vi "NMRFMTCP5.vi"() -> ()   [LabVIEW 2013]
uses:
  <vilib>/Analysis/2dsp.llb/Power Spectrum (DBL).vi
  kleinjan/MKS/Global - Pressure & Flow.vi
  <vilib>/Analysis/NI_AALBase.lvlib
  <vilib>/Analysis/NI_AALPro.lvlib
panel:
  out "initphase":dbl=2.08 format="%#_13g"
  out "inittune":dbl=1.244 format="%#_13g"
  in  "Save Tune":bool
  in  "Tune?":bool
  out "Date / Time":string="12/5/2017 4:21:17 PM"
  in  "Stop Run":bool=TRUE
  out "He readback":bool
  in  "Prompt?":bool
  out "He temp (K)":sgl=2.13326 format="%.3f"
  out "He press (torr)":sgl=33.89 format="%.3f"
  in  "NMR Channel Select":string(combo)="Tune2.csv"
  out "Color Box":u32(colorbox)=16775210
  out "Measurement":enum16{"TEQ", "POL", "QCV"}(ring)
  in  "VME IP Address":string="192.168.0.4"
  out "FFT Vrms":dbl[](graph)=[0.00665461346633416, 0.0013184205958180774, 0.00032493347048972255, 0.00014777056763622272, 9.381274661705268e-05, 5.694492256043897e-05, 2.4602515151070093e-05, 2.4735928736174615e-05, 1.7238804666774456e-05, 1.8474256556130103e-05, 3.88140821584203e-06, 1.2602440301653875e-05, 8.328027067854474e-06, 9.714098656211597e-06, 9.591073826282002e-06, 1.8400610475153133e-06, 3.891822160858666e-06, 7.42860213832651e-07, 4.960531568911141e-06, 1.0357752920077204e-05, 8.821106198975682e-06, 4.297248862721329e-06, 6.756736241898357e-06, 1.1507829286001889e-05, 6.285430593231241e-06, 5.699497906089993e-06, 4.826883317592869e-06, 1.0954894980259898e-05, 8.548451061857287e-06, 8.288312118460071e-07, 3.496252158688967e-06, 4.446519758691104e-06, 1.1272471497109705e-06, 2.984287855648866e-06, 4.4013212799680506e-06, 2.7233378655836314e-06, 8.028051828202549e-06, 2.7179961404271994e-06, 2.741222097162825e-06, 8.272000128623847e-06, 5.062564520990176e-06, 5.342721918389221e-06, 4.655150514690805e-06, 3.7370639785257395e-06, 2.136800574890996e-06, 1.8266511330512507e-06, 1.284347857617383e-06, 2.0013558699868966e-06, 1.2042755969189114e-06, 6.058284222290214e-06, 7.389298504405541e-06, 2.77971188428063e-06, 7.697014337872333e-06, 4.09073583086401e-06, 3.1016991758581816e-06, 5.282645474294868e-07, 3.246106814596551e-06, 1.5964327844448069e-06, 3.2408118302431348e-06, 1.9033736338368444e-06, 6.683740481872343e-06, 2.6688168177704896e-06, 1.8040110478604363e-06, 5.689652571752047e-07, 4.566365523818322e-06, 7.67651980126649e-06, 3.6261391438622403e-06, 1.962113938019778e-06, 1.9575774542411484e-06, 6.113330203835039e-06, 4.837593307405045e-06, 1.5646329065944149e-06, 1.9642799364610824e-06, 5.344757267984994e-06, 1.4903732944971783e-06, 2.3253986011212398e-06, 3.505294515533926e-06, 1.2861248933475453e-06, 3.1756847203363983e-06, 5.210539488954998e-06, 5.873764257939144e-06, 1.488838318327932e-06, 3.4258096560470588e-06, 4.6561579367461355e-06, 3.3604761794694807e-06, 5.166120910958792e-06, 4.852422673140418e-06, 6.413144484541961e-06, 2.3873635432332113e-06, 4.815191295361827e-06, 4.599370623864332e-06, 4.533502118577405e-06, 4.251902968067585e-06, 1.1589988767519234e-06, 2.3203344894473095e-07, 4.066434795829476e-06, 3.46145032312765e-06, 3.2547198313791895e-06, 2.1219983709150387e-06, 4.495545878631818e-06, 3.110572503955211e-07, 1.589264311064526e-06, 3.3006546489564546e-06, 3.239107109046435e-06, 1.956587615390749e-06, 1.0821609125242872e-06, 4.18172944578455e-06, 3.4672825501217612e-06, 3.0604596728264873e-06, 2.249802101656082e-06, 3.6396234355254457e-06, 1.9148250175480704e-06, 6.100574262898342e-06, 2.040562898958206e-06, 3.681543145664905e-06, 6.36570977326168e-06, 3.978270510621126e-06, 2.9167261060330305e-06, 4.596371371759104e-06, 1.7082086474587407e-06, 1.0983887595677434e-06, 1.6801012803857932e-06, 1.8127834158020698e-06, 4.439505513519553e-06, 1.6592215036724682e-06, 2.5343701898196556e-06, 6.407230283423339e-06, 2.878137385486302e-06, 1.0359403307825742e-06, 3.401981562355416e-06, 4.492298826850195e-06, 4.244045593799213e-06, 2.4547652511595895e-06, 2.287980497906362e-06, 4.064951112754048e-06, 1.0150896867566275e-05, 5.111642196581524e-06, 2.7553627360277643e-06, 5.09313899121079e-07, 5.768699698084646e-06, 3.2661863048088682e-06, 5.576911536051898e-06, 1.3992030895115723e-06, 5.793480137064482e-07, 4.167273754327372e-06, 2.803767211933649e-06, 1.290492108720642e-06, 1.4073374274672208e-06, 2.2326186185191207e-06, 2.361435359052297e-06, 1.1075042044185725e-06, 9.822428126647478e-07, 1.4402015890510517e-06, 3.4799861239118846e-06, 6.876662204989774e-07, 2.9528766955207207e-06, 3.987038034312176e-06, 2.4223930611358374e-06, 2.4859113073777655e-06, 2.676948548044152e-06, 3.001197081641741e-06, 1.3437660563498952e-06, 4.530463234261475e-06, 3.5418577344012663e-06, 9.285218882268811e-07, 2.448991731608343e-06, 4.237615365541793e-06, 9.437753499711396e-06, 4.733601144522179e-06, 1.1993912833596027e-06, 4.592206510692074e-06, 1.6445086805399158e-06, 2.28625361595349e-06, 2.7657675123967644e-06, 4.727937271980666e-06, 1.1243035877642484e-06, 2.963405459320666e-06, 2.4221501912349967e-06, 4.3573020759701795e-06, 6.067249298625184e-06, 4.689337884831793e-06, 1.5356012824001038e-06, 4.493628958545829e-06, 2.750405264990747e-06, 1.803652857072422e-06, 5.477945487956627e-06, 4.241114523214695e-06, 3.110895691004747e-06, 4.4944025519747775e-06, 1.9660519605861145e-06, 3.642406557905753e-06, 3.6774228456584596e-06, 1.6639882217832455e-06, 6.260045262480856e-07, 4.334327770598918e-06, 5.214873834167074e-06, 1.730017114321754e-06, 1.93737641122103e-06, 3.517495286731861e-06, 1.7057836116701932e-06, 3.185318567505982e-06, 3.185318567505982e-06, 1.7057836116701932e-06, 3.517495286731861e-06, 1.93737641122103e-06, 1.730017114321754e-06, 5.214873834167074e-06, 4.334327770598918e-06, 6.260045262480856e-07, 1.6639882217832455e-06, 3.6774228456584596e-06, 3.642406557905753e-06, 1.9660519605861145e-06, 4.4944025519747775e-06, 3.110895691004747e-06, 4.241114523214695e-06, 5.477945487956627e-06, 1.803652857072422e-06, 2.750405264990747e-06, 4.493628958545829e-06, 1.5356012824001038e-06, 4.689337884831793e-06, 6.067249298625184e-06, 4.3573020759701795e-06, 2.4221501912349967e-06, 2.963405459320666e-06, 1.1243035877642484e-06, 4.727937271980666e-06, 2.7657675123967644e-06, 2.28625361595349e-06, 1.6445086805399158e-06, 4.592206510692074e-06, 1.1993912833596027e-06, 4.733601144522179e-06, 9.437753499711396e-06, 4.237615365541793e-06, 2.448991731608343e-06, 9.285218882268811e-07, 3.5418577344012663e-06, 4.530463234261475e-06, 1.3437660563498952e-06, 3.001197081641741e-06, 2.676948548044152e-06, 2.4859113073777655e-06, 2.4223930611358374e-06, 3.987038034312176e-06, 2.9528766955207207e-06, 6.876662204989774e-07, 3.4799861239118846e-06, 1.4402015890510517e-06, 9.822428126647478e-07, 1.1075042044185725e-06, 2.361435359052297e-06, 2.2326186185191207e-06, 1.4073374274672208e-06, 1.290492108720642e-06, 2.803767211933649e-06, 4.167273754327372e-06, 5.793480137064482e-07, 1.3992030895115723e-06, 5.576911536051898e-06, 3.2661863048088682e-06, 5.768699698084646e-06, 5.09313899121079e-07, 2.7553627360277643e-06, 5.111642196581524e-06, 1.0150896867566275e-05, 4.064951112754048e-06, 2.287980497906362e-06, 2.4547652511595895e-06, 4.244045593799213e-06, 4.492298826850195e-06, 3.401981562355416e-06, 1.0359403307825742e-06, 2.878137385486302e-06, 6.407230283423339e-06, 2.5343701898196556e-06, 1.6592215036724682e-06, 4.439505513519553e-06, 1.8127834158020698e-06, 1.6801012803857932e-06, 1.0983887595677434e-06, 1.7082086474587407e-06, 4.596371371759104e-06, 2.9167261060330305e-06, 3.978270510621126e-06, 6.36570977326168e-06, 3.681543145664905e-06, 2.040562898958206e-06, 6.100574262898342e-06, 1.9148250175480704e-06, 3.6396234355254457e-06, 2.249802101656082e-06, 3.0604596728264873e-06, 3.4672825501217612e-06, 4.18172944578455e-06, 1.0821609125242872e-06, 1.956587615390749e-06, 3.239107109046435e-06, 3.3006546489564546e-06, 1.589264311064526e-06, 3.110572503955211e-07, 4.495545878631818e-06, 2.1219983709150387e-06, 3.2547198313791895e-06, 3.46145032312765e-06, 4.066434795829476e-06, 2.3203344894473095e-07, 1.1589988767519234e-06, 4.251902968067585e-06, 4.533502118577405e-06, 4.599370623864332e-06, 4.815191295361827e-06, 2.3873635432332113e-06, 6.413144484541961e-06, 4.852422673140418e-06, 5.166120910958792e-06, 3.3604761794694807e-06, 4.6561579367461355e-06, 3.4258096560470588e-06, 1.488838318327932e-06, 5.873764257939144e-06, 5.210539488954998e-06, 3.1756847203363983e-06, 1.2861248933475453e-06, 3.505294515533926e-06, 2.3253986011212398e-06, 1.4903732944971783e-06, 5.344757267984994e-06, 1.9642799364610824e-06, 1.5646329065944149e-06, 4.837593307405045e-06, 6.113330203835039e-06, 1.9575774542411484e-06, 1.962113938019778e-06, 3.6261391438622403e-06, 7.67651980126649e-06, 4.566365523818322e-06, 5.689652571752047e-07, 1.8040110478604363e-06, 2.6688168177704896e-06, 6.683740481872343e-06, 1.9033736338368444e-06, 3.2408118302431348e-06, 1.5964327844448069e-06, 3.246106814596551e-06, 5.282645474294868e-07, 3.1016991758581816e-06, 4.09073583086401e-06, 7.697014337872333e-06, 2.77971188428063e-06, 7.389298504405541e-06, 6.058284222290214e-06, 1.2042755969189114e-06, 2.0013558699868966e-06, 1.284347857617383e-06, 1.8266511330512507e-06, 2.136800574890996e-06, 3.7370639785257395e-06, 4.655150514690805e-06, 5.342721918389221e-06, 5.062564520990176e-06, 8.272000128623847e-06, 2.741222097162825e-06, 2.7179961404271994e-06, 8.028051828202549e-06, 2.7233378655836314e-06, 4.4013212799680506e-06, 2.984287855648866e-06, 1.1272471497109705e-06, 4.446519758691104e-06, 3.496252158688967e-06, 8.288312118460071e-07, 8.548451061857287e-06, 1.0954894980259898e-05, 4.826883317592869e-06, 5.699497906089993e-06, 6.285430593231241e-06, 1.1507829286001889e-05, 6.756736241898357e-06, 4.297248862721329e-06, 8.821106198975682e-06, 1.0357752920077204e-05, 4.960531568911141e-06, 7.42860213832651e-07, 3.891822160858666e-06, 1.8400610475153133e-06, 9.591073826282002e-06, 9.714098656211597e-06, 8.328027067854474e-06, 1.2602440301653875e-05, 3.88140821584203e-06, 1.8474256556130103e-05, 1.7238804666774456e-05, 2.4735928736174615e-05, 2.4602515151070093e-05, 5.694492256043897e-05, 9.381274661705268e-05, 0.00014777056763622272, 0.00032493347048972255, 0.0013184205958180774]
  out "Raw NMR Graph / Ave":cluster{dbl, "Step Width (MHz)":dbl, dbl[][]}(graph)={212.6, "Step Width (MHz)"=0.002, []}
  in  "R&S GPIB Addr (28)":refnum<visa-resource-name>="GPIB1::28::INSTR"
  out "Pedestal (V)":dbl=0.007879166666666666 format="%_2g"
  in  "Open Global Panel":bool
  out "Peak center (MHz)":sgl=212.61032 format="%.3f"
  out "Telnet error out":errorcluster
  out "+3.3V supply":dbl=3.294 format="%_4g"
  out "Temp (C)":dbl=25.0 format="%_4g"
  out "RF level OK":bool=TRUE
  out "Peak area (V-MHz)":sgl=-0.97693336 format="%.5f"
  out "# Good Spectra":i32=1000
  out "Pedestal volts OK":bool=TRUE
  out "Sweep #":i32=88
  out "1st Sweep":bool
  out "ADC volts OK":bool=TRUE
  out "Peak Height Distribution":cluster{"Y":dbl[], "Y":dbl[]}[](graph)=[{"Y"=[0.003985987500000001, 0.0039929625000000015, 0.003999937500000002, 0.004006912500000002, 0.004013887500000001, 0.0040208625000000015, 0.004027837500000002, 0.004034812500000002, 0.004041787500000001, 0.0040487625000000015, 0.004055737500000002, 0.004062712500000002, 0.004069687500000001, 0.0040766625000000015, 0.004083637500000002, 0.004090612500000001, 0.004097587500000001, 0.0041045625000000014, 0.004111537500000002, 0.004118512500000001, 0.004125487500000001, 0.004132462500000001, 0.004139437500000002, 0.004146412500000001, 0.004153387500000001, 0.004160362500000001, 0.004167337500000002, 0.004174312500000001, 0.004181287500000001, 0.004188262500000001, 0.004195237500000002, 0.004202212500000001, 0.004209187500000001, 0.004216162500000001, 0.0042231375000000015, 0.004230112500000001, 0.004237087500000001, 0.004244062500000001, 0.004251037500000001, 0.004258012500000001, 0.004264987500000001, 0.004271962500000001, 0.004278937500000001, 0.004285912500000001, 0.004292887500000001, 0.004299862500000001, 0.004306837500000001, 0.004313812500000001, 0.004320787500000001, 0.004327762500000001, 0.004334737500000001, 0.004341712500000001, 0.004348687500000001, 0.004355662500000001, 0.0043626375000000005, 0.004369612500000001, 0.004376587500000001, 0.004383562500000001, 0.0043905375000000005, 0.004397512500000001, 0.004404487500000001, 0.004411462500000001, 0.0044184375000000005, 0.004425412500000001, 0.004432387500000001, 0.0044393625, 0.0044463375000000005, 0.004453312500000001, 0.004460287500000001, 0.0044672625, 0.0044742375000000004, 0.004481212500000001, 0.004488187500000001, 0.0044951625, 0.0045021375, 0.004509112500000001, 0.004516087500000001, 0.0045230625, 0.0045300375, 0.004537012500000001, 0.004543987500000001, 0.0045509625, 0.0045579375, 0.004564912500000001, 0.004571887500000001, 0.0045788625, 0.0045858375, 0.0045928125000000005, 0.004599787500000001, 0.0046067625, 0.0046137375, 0.0046207125000000005, 0.0046276875, 0.0046346625, 0.0046416375, 0.0046486125000000005, 0.0046555875, 0.0046625625, 0.0046695375, 0.0046765125000000005], "Y"=[1.0, 0.0, 0.0, 0.0, 0.0, 0.0, 0.0, 0.0, 2.0, 1.0, 0.0, 0.0, 0.0, 1.0, 4.0, 3.0, 3.0, 1.0, 0.0, 8.0, 2.0, 8.0, 8.0, 3.0, 2.0, 12.0, 12.0, 12.0, 2.0, 17.0, 13.0, 11.0, 11.0, 17.0, 19.0, 14.0, 17.0, 24.0, 13.0, 17.0, 14.0, 22.0, 21.0, 25.0, 26.0, 26.0, 23.0, 21.0, 29.0, 18.0, 25.0, 31.0, 24.0, 45.0, 24.0, 20.0, 29.0, 22.0, 19.0, 23.0, 17.0, 8.0, 13.0, 18.0, 24.0, 12.0, 22.0, 18.0, 8.0, 8.0, 10.0, 9.0, 13.0, 8.0, 8.0, 6.0, 5.0, 5.0, 4.0, 4.0, 4.0, 8.0, 3.0, 5.0, 3.0, 1.0, 1.0, 1.0, 3.0, 1.0, 1.0, 0.0, 1.0, 0.0, 0.0, 1.0, 0.0, 1.0, 0.0, 1.0]}]
  out "S/N":dbl=39.7281597738682 format="%_3g"
  out "Peak mean (V)":dbl=0.004333396666666667 format="%_3g"
  out "Pedestal Diff (V)":sgl=-0.00025166667 format="%.4f"
  out "Peak amp (V)":sgl=0.0031208333 format="%.4f"
  out "SMT error out":errorcluster
  out "Peak RMS (mV)":dbl=0.10907619913261185 format="%.3f"
  # "E1039 NMR Panel"
  # "Results"
  # "A\nv\ne\nr\na\ng\ne\ns"
  # "S\nw\ne\ne\np"
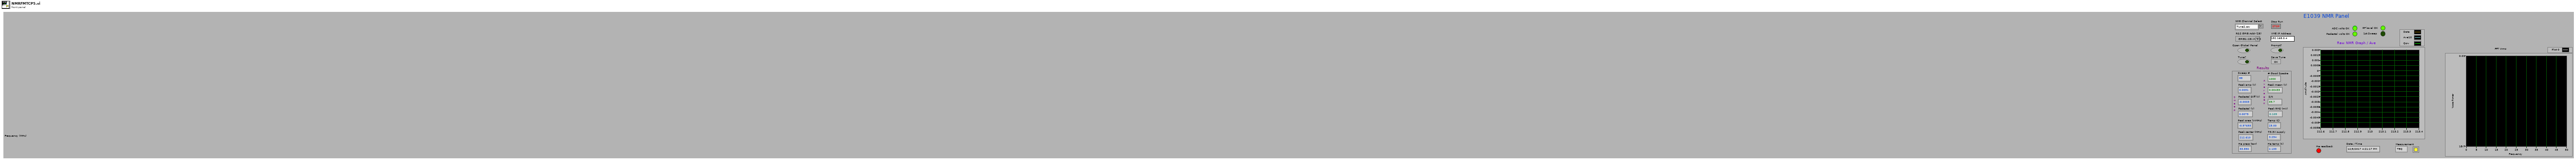
[diagram p1: front panel]
types:
  T1 = enum32{"Invalid", "Standard", "Closed", "Hidden", "Minimized", "Maximized"}
  T2 = enum32{"Bad", "Idle", "Run top level", "Running"}
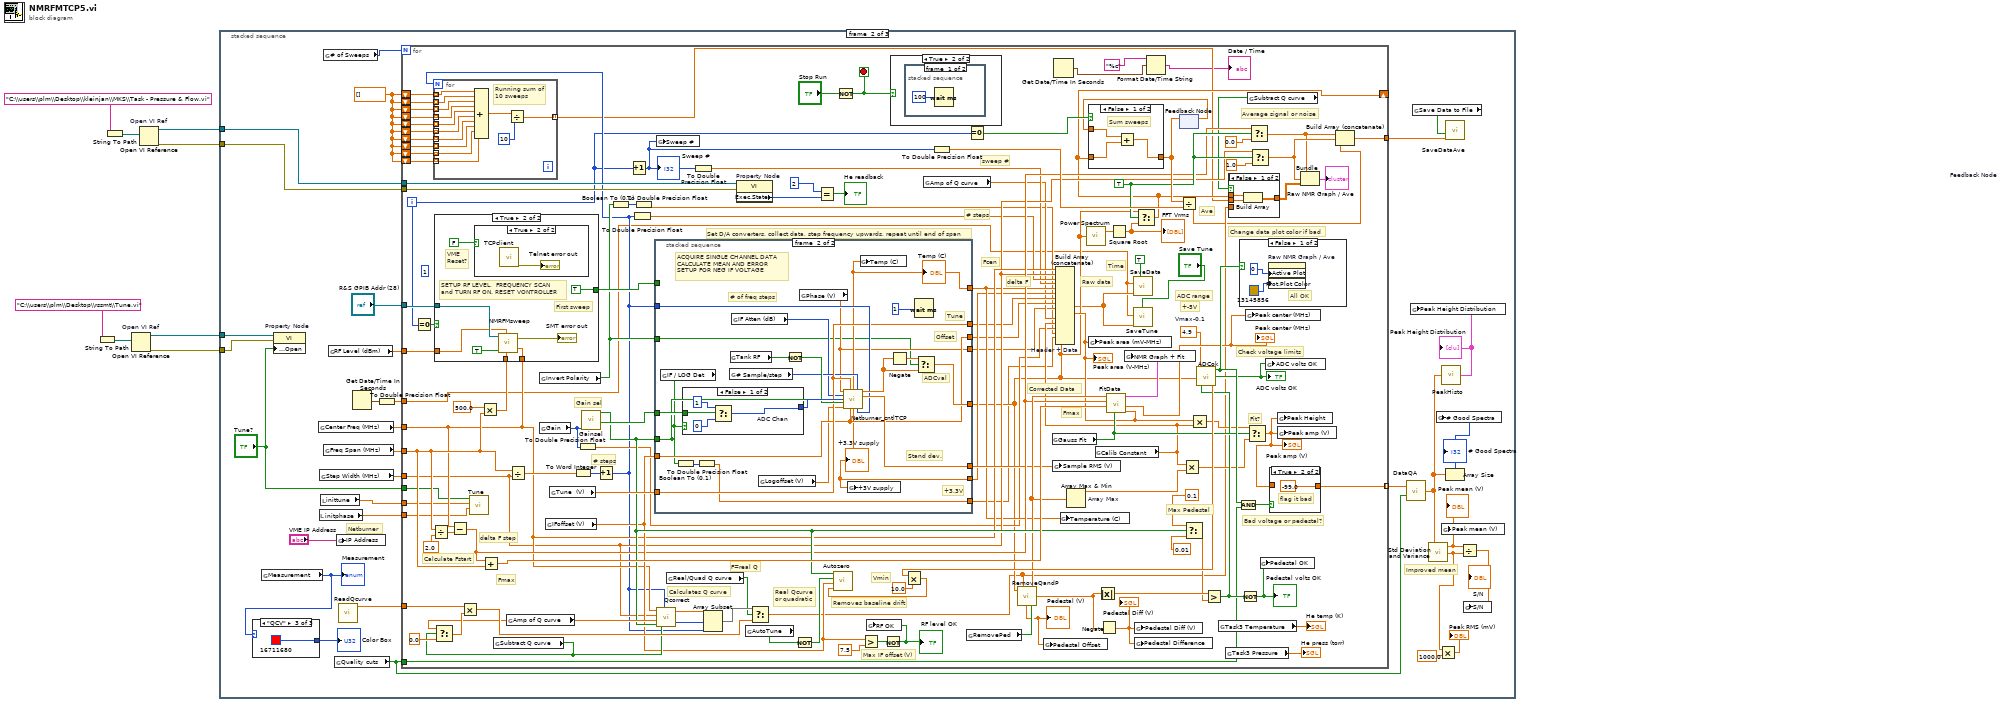
[diagram p0: block diagram]
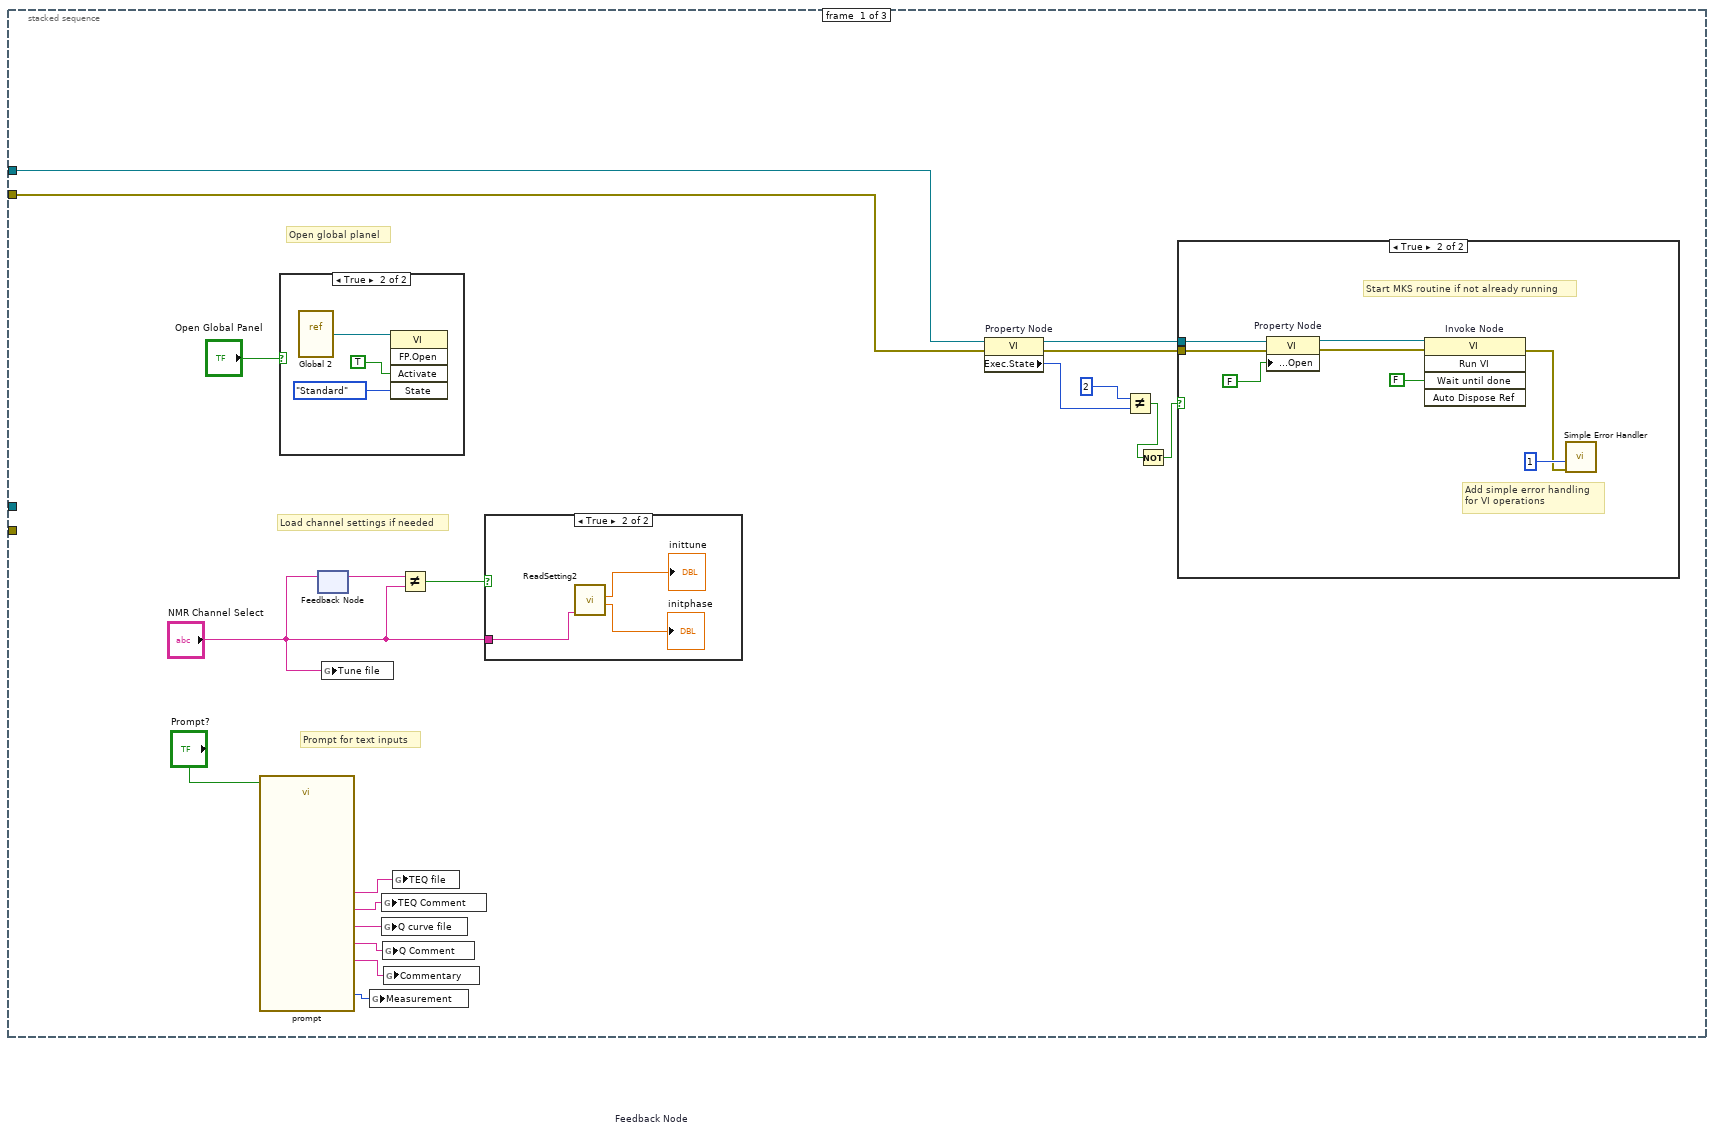
[diagram p2: hidden frame]
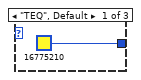
[diagram p6: hidden frame]
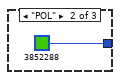
[diagram p7: hidden frame]
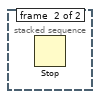
[diagram p9: hidden frame]
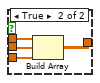
[diagram p10: hidden frame]
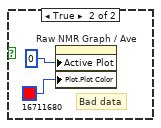
[diagram p12: hidden frame]
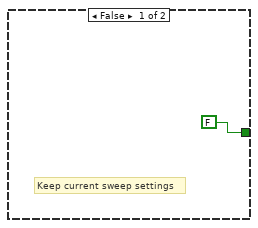
[diagram p14: hidden frame]
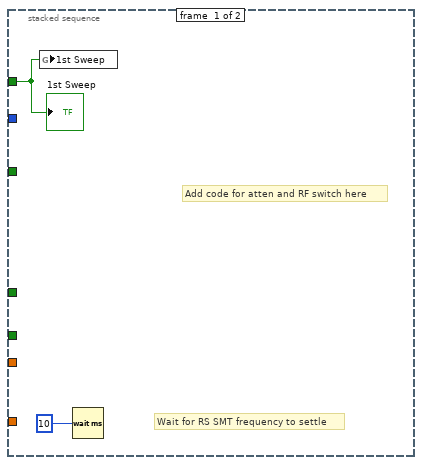
[diagram p16: hidden frame]
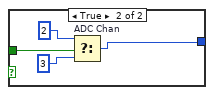
[diagram p17: hidden frame]
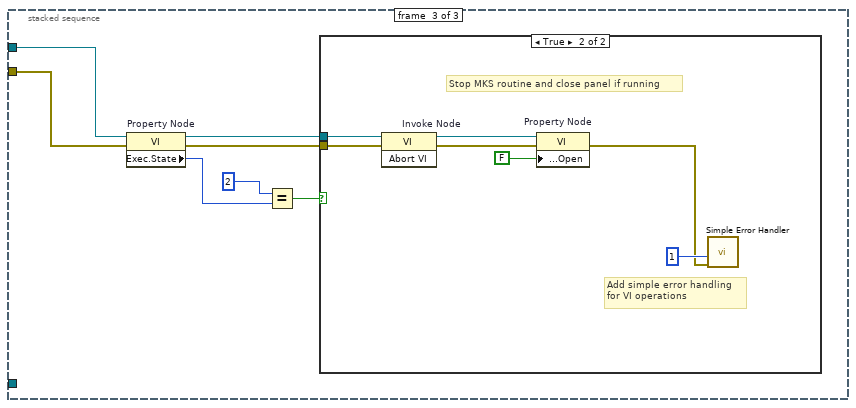
[diagram p18: hidden frame]
diagram:
  n1 = String To Path(string="C:\\users\\plm\\Desktop\\rssmt\\Tune.vi") -> (path=w4:path)
  n2 = String To Path(string="C:\\users\\plm\\Desktop\\kleinjan\\MKS\\Task - Pressure & Flow.vi") -> (path=w8:path)
  n3 = Open VI Reference "Open VI Ref"(vi path=w4) -> (vi reference=w2:refnum<vi>, error out=w1:errorcluster)  [unwired: 5 in]
  n4 = Open VI Reference "Open VI Ref"(vi path=w8) -> (vi reference=w5:refnum<vi>, error out=w6:errorcluster)  [unwired: 5 in]
  n5 = stacked-sequence {
    tunnel: w5 -> [w12 w49 w282]
    tunnel: w6 -> [w11 w48 w281]
    tunnel: w2 -> [_ w42 _]
    tunnel: w1 -> [_ w46 _]
    frame #0 {
      # "Prompt for text inputs"
      # "Load channel settings if needed"
      # "Open global planel"
      n6 = call "prompt.vi"("Enable"="Prompt?") -> ("Measurement"=w25:enum16{"TEQ", "POL", "QCV"}, "Run comment"=w24:string, "Q curve comment"=w23:string, "Q curve file"=w22:string, "TE Comment"=w21:string, "TE peak file"=w20:string)  [unwired: 11 in, 2 out]
      n7 = case shown="True" "Open Global Panel" {
        frame False {
        }
        frame True {
          n8 = vi-ref "Global 2.vi"() -> (w41:refnum<vi>)
          n9 = invoke class="VI" method="FP.Open"(reference=w41, "Activate"=TRUE, "State"=T1."Standard") -> ()  [unwired: 2 in, 5 out]
        }
      }
      n10 = feedback #1 "Feedback Node"() -> (w19:string)  [unwired: 1 in]
      n11 = feedback-in #1("NMR Channel Select") -> ()
      n12 = global write "Global 2.vi" "Tune file"("NMR Channel Select") -> ()
      n13 = global write "Global 2.vi" "Measurement"(w25) -> ()
      n14 = global write "Global 2.vi" "TEQ Comment"(w21) -> ()
      n15 = global write "Global 2.vi" "Q curve file"(w22) -> ()
      n16 = global write "Global 2.vi" "Q Comment"(w23) -> ()
      n17 = global write "Global 2.vi" "Commentary"(w24) -> ()
      n18 = global write "Global 2.vi" "TEQ file"(w20) -> ()
      n19 = Not Equal?(x=w19, y="NMR Channel Select") -> (x != y?=w18:bool)
      n20 = case shown="True" w18 {
        tunnel: "NMR Channel Select" -> [_ w38]
        frame False {
        }
        frame True {
          n21 = call "ReadSetting2.vi"("Data Filename"=w38) -> ("Phase"=→"initphase":dbl, "Tune"=→"inittune":dbl)  [unwired: 1 out]
        }
      }
      n22 = property on="Property Node" class="VI"(reference=w12, error in=w11) -> (reference out=w14:refnum<vi>, error out=w13:errorcluster, "Exec.State"=w15:T2)
      n23 = Not Equal?(x=2, y=w15) -> (x != y?=w10:bool)
      n24 = Not(x=w10) -> (.not. x?=w9:bool)
      n25 = case shown="True" w9 {
        tunnel: w14 -> [_ w32]
        tunnel: w13 -> [_ w31]
        frame False {
        }
        frame True {
          # "Start MKS routine if not already running"
          # "Add simple error handling\nfor VI operations"
          n26 = property on="Property Node" class="VI"(reference=w32, error in=w31, "Front Panel Window:Open"=FALSE ("Front Panel.Open")) -> (reference out=w30:refnum<vi>, error out=w29:errorcluster)
          n27 = invoke on="Invoke Node" class="VI" method="Run VI"(reference=w30, error in=w29, "Wait until done"=FALSE) -> (error out=w33:errorcluster)  [unwired: 2 in, 4 out]
          n28 = call <vilib>:"Simple Error Handler.vi"("type of dialog (OK msg:1)"=1, "error in (no error)"=w33) -> ()  [unwired: 3 in, 5 out]
        }
      }
    }
    frame #1 {
      w47 = dbl[] []
      # "Netburner"
      # "Improved mean"
      n29 = global read "Global 2.vi" "Measurement"() -> (w51:enum16{"TEQ", "POL", "QCV"})
      "Measurement" <- w51
      n30 = case shown="\"QCV\"" w51 {
        tunnel: [u32 16775210 ("Color Box 2") u32 3852288 ("Color Box 2") u32 16711680 ("Color Box 2")] -> w50
        frame "TEQ", Default {
        }
        frame "POL" {
        }
        frame "QCV" {
        }
      }
      "Color Box" <- w50
      n31 = property on="Property Node" class="VI"(reference=w42, error in=w46, "Front Panel Window:Open"="Tune?") -> ()  [unwired: 2 out]
      n32 = global read "Global 2.vi" "Center Freq (MHz)"() -> (w68:dbl)
      n33 = local read "initphase"() -> (w43:dbl)
      n34 = global read "Global 2.vi" "Step Width (MHz)"() -> (w66:dbl)
      n35 = local read "inittune"() -> (w44:dbl)
      n36 = global read "Global 2.vi" "# of Sweeps"() -> (w70:i32)
      n37 = global read "Global 2.vi" "Freq Span (MHz)"() -> (w67:dbl)
      n38 = global read "Global 2.vi" "RF Level (dBm)"() -> (w69:dbl)
      n39 = global read "Global 2.vi" "Quality cuts"() -> (w65:bool)
      n40 = global write "Global 2.vi" "IP Address"("VME IP Address") -> ()
      n41 = call "ReadQcurve.vi"() -> ("Array"=w56:dbl[])  [unwired: 2 in]
      n42 = Get Date/Time In Seconds() -> (seconds since 1Jan1904=w71:timestamp)
      n43 = To Double Precision Float(number=w71) -> (double precision float=w57:dbl)
      n44 = for {
        N: w70 -> [_]
        tunnel: [w198] -> w73 mode=indexing
        tunnel: w65 -> [w161]
        tunnel: w68 -> [w135]
        tunnel: w67 -> [w147]
        tunnel: w66 -> [w134]
        tunnel: "R&S GPIB Addr (28)" -> [w194]
        tunnel: w69 -> [w193]
        tunnel: w57 -> [w81]
        tunnel: w56 -> [w186]
        tunnel: [w151] -> w59
        tunnel: w49 -> [w108]
        tunnel: w48 -> [w107]
        shift-right: [w100] -> _
        shift-left: w47 -> [w99]
        shift-left: w47 -> [w90]
        shift-left: w47 -> [w98]
        shift-left: w47 -> [w97]
        shift-left: w47 -> [w96]
        shift-left: w47 -> [w95]
        shift-left: w47 -> [w94]
        shift-left: w47 -> [w93]
        shift-left: w47 -> [w92]
        shift-left: w47 -> [w91]
        tunnel: "Tune?" -> [w83]
        tunnel: w44 -> [w79]
        tunnel: w43 -> [w78]
        i -> [w88]
        stop <- w77 stop-if-true
        (unwired) 1
        w140 = TRUE
        w156 = 4.9  # Vmax-0.1
        # "Average signal or noise"
        # "Check voltage limits"
        # "Ave"
        # "Max Pedestal"
        # "Gain sel"
        # "F=real Q"
        # "Real Qcurve\nor quadratic"
        # "+-5V"
        # "Change data plot color if bad"
        # "Max IF offset (V)"
        # "Fmax"
        # "Fit?"
        # "Fmax"
        # "Time"
        # "Vmin"
        # "Raw data"
        # "Corrected Data"
        # "Fcen"
        # "delta F"
        # "# steps"
        # "ADC range"
        # "sweep #"
        # "Set D/A converters, collect data, step frequency upwards, repeat until end of span"
        # "Calculates Q curve"
        # "Removes baseline drift"
        # "Bad voltage or pedestal?"
        # "# steps"
        # "Calculate Fstart"
        # "delta F step"
        n45 = Equal To 0?(x=w88) -> (x = 0?=w200:bool)
        n46 = Divide(x=w147, y=sgl 2.0) -> (x/y=w204:dbl)
        n47 = Subtract(x=w135, y=w204) -> (x-y=w138:dbl)
        n48 = call "Tune.vi"("Init Phase V"=w78, "Init Tune V"=w79, "Tune"=w83) -> ()  [unwired: 9 in]
        n49 = Multiply(x=500.0, y=w147) -> (x*y=w146:dbl)
        n50 = case shown="True" w200 {
          tunnel: w135 -> [_ w245]
          tunnel: w146 -> [_ w246]
          tunnel: [FALSE TRUE] -> w199
          tunnel: w194 -> [_ w242]
          tunnel: w193 -> [_ w241]
          frame False {
            # "Keep current sweep settings"
          }
          frame True {
            # "VME\nReset?"
            # "First sweep"
            # "SETUP RF LEVEL,  FREQUENCY SCAN\nand TURN RF ON. RESET VONTROLLER"
            n51 = case shown="True" FALSE {
              frame False {
              }
              frame True {
                n52 = call "TCPclient.vi"() -> ("Telnet error"=→"Telnet error out":errorcluster)  [unwired: 4 in, 3 out]
              }
            }
            n53 = call "NMRFMsweep.vi"("Center Freq (MHz)"=w245, "Freq Span (kHz)"=w246, "RF Level (dBm)"=w241, "Program"=TRUE, "GPIB Addr (28)"=w242) -> ("error out"=→"SMT error out":errorcluster)  [unwired: 2 in]
          }
        }
        n54 = Add(x=w138, y=w147) -> (x+y=w190:dbl)
        n55 = global read "Global 2.vi" "Subtract Q curve"() -> (w177:bool)
        n56 = global read "Global 2.vi" "Amp of Q curve"() -> (w178:dbl)
        n57 = Select(t=w178, s=w177, f=0.0) -> (s? t:f=w183:dbl)
        n58 = Multiply(x=w186, y=w183) -> (x*y=w185:dbl[])
        n59 = Divide(x=w147, y=w134) -> (x/y=w206:dbl)
        n60 = global read "Global 2.vi" "Invert Polarity"() -> (w116:bool)
        n61 = global read "Global 2.vi" "Gain"() -> (w121:enum16{"LOW", "HI", "MAX"})
        n62 = global read "Global 2.vi" "IFoffset (V)"() -> (w150:dbl)
        n63 = global read "Global 2.vi" "Tune  (V)"() -> (w179:dbl)
        n64 = To Word Integer(number=w206) -> (16bit integer=w203:i16)
        n65 = To Double Precision Float(number=w121) -> (double precision float=w120:dbl)
        n66 = call "Gainsel.vi"("Gain"=w121) -> ("LO"=w153:bool, "MAX"=w152:bool)  [unwired: 1 out]
        n67 = Increment(x=w203) -> (x+1=w89:i16)
        n68 = for {
          N: w89 -> [_]
          tunnel: w99 -> [w211] mode=indexing
          tunnel: w98 -> [w219] mode=indexing
          tunnel: w97 -> [w218] mode=indexing
          tunnel: w96 -> [w217] mode=indexing
          tunnel: w95 -> [w216] mode=indexing
          tunnel: w94 -> [w215] mode=indexing
          tunnel: w93 -> [w214] mode=indexing
          tunnel: w92 -> [w213] mode=indexing
          tunnel: w91 -> [w212] mode=indexing
          tunnel: w90 -> [w220] mode=indexing
          tunnel: [w208] -> w87 mode=indexing
          # "Running sum of 10 sweeps"
          n69 = Compound Arithmetic op=ADD(w211, w220, w219, w218, w217, w216, w215, w214, w213, w212) -> (w209:dbl)
          n70 = Divide(x=w209, y=10) -> (x/y=w208:dbl)
        }
        n71 = Boolean To (0,1)(Boolean=w116) -> (0, 1=w117:i16)
        n72 = Increment(x=w88) -> (x+1=w159:i32)
        "Sweep #" <- w159
        n73 = To Double Precision Float(number=w89) -> (double precision float=w133:dbl)
        n74 = To Double Precision Float(number=w117) -> (double precision float=w115:dbl)
        n75 = stacked-sequence {
          tunnel: [_ w267] -> w136
          tunnel: [_ w271] -> w119
          tunnel: w89 -> [_ w265]
          tunnel: w150 -> [_ w262]
          tunnel: w153 -> [_ w269]
          tunnel: w199 -> [w248 _]
          tunnel: w179 -> [_ w263]
          tunnel: [_ w256] -> w131
          tunnel: [_ w255] -> w130
          tunnel: [_ w263] -> w129
          tunnel: [_ w262] -> w128
          tunnel: [_ w261] -> _
          tunnel: w152 -> [_ w261]
          tunnel: [_ w254] -> w118
          tunnel: w116 -> [_ w253]
          tunnel: [_ w250] -> w114
          frame #0 {
            # "Add code for atten and RF switch here"
            # "Wait for RS SMT frequency to settle"
            n76 = global write "Global 2.vi" "1st Sweep"(w248) -> ()
            n77 = Wait (ms)(milliseconds to wait=10) -> ()  [unwired: 1 out]
            "1st Sweep" <- w248
          }
          frame #1 {
            # "+3.3V"
            # "Offset"
            # "Tune"
            # "Stand dev."
            # "ADCval"
            # "ACQUIRE SINGLE CHANNEL DATA\nCALCULATE MEAN AND ERROR\nSETUP FOR NEG IF VOLTAGE"
            # "# of freq steps"
            n78 = global read "Global 2.vi" "IF / LOG Det"() -> (w252:bool)
            n79 = Boolean To (0,1)(Boolean=w252) -> (0, 1=w251:i16)
            n80 = case shown="False" w252 {
              tunnel: w269 -> [w276 w277]
              tunnel: [w273 w278] -> w266
              frame False {
                n81 = Select "ADC Chan"(t=1, s=w276, f=0) -> (s? t:f=w273:i32)
              }
              frame True {
                n82 = Select "ADC Chan"(t=2, s=w277, f=3) -> (s? t:f=w278:i32)
              }
            }
            n83 = To Double Precision Float(number=w251) -> (double precision float=w250:dbl)
            n84 = global read "Global 2.vi" "# Sample/step"() -> (w258:i32)
            n85 = global read "Global 2.vi" "Tank RF"() -> (w259:bool)
            n86 = global read "Global 2.vi" "IF Atten (dB)"() -> (w257:i8)
            n87 = global read "Global 2.vi" "Logoffset (V)"() -> (w260:dbl)
            n88 = Not(x=w259) -> (.not. x?=w264:bool)
            n89 = global read "Global 2.vi" "Phase (V)"() -> (w254:dbl)
            n90 = call "Netburner_cntlTCP.vi"("Phase Volt"=w254, "Tune Volt"=w263, "# Data"=w258, "IF Atten (dB)"=w257, "NMR ADC"=w266, "Hi Gain"=w261, "Tank RF"=w264, "LogOff Volt"=w260, "IFOff Volt"=w262, "# f steps"=w265) -> ("Temp (C)"=w256:dbl, "ADC value"=w268:dbl[], "ADC Std Dev"=w267:dbl, "Volts"=w255:dbl)  [unwired: 2 out]
            "Temp (C)" <- w256
            "+3.3V supply" <- w255
            n91 = global write "Global 2.vi" "+3V supply"(w255) -> ()
            n92 = global write "Global 2.vi" "Temp (C)"(w256) -> ()
            n93 = Negate(x=w268) -> (-x=w270:dbl[])
            n94 = Wait (ms)(milliseconds to wait=1) -> ()  [unwired: 1 out]
            n95 = Select(t=w270, s=w253, f=w268) -> (s? t:f=w271:dbl[])
          }
        }
        n96 = global write "Global 2.vi" "Sweep #"(w159) -> ()
        n97 = call "Qcorrect.vi"("Subtract Q curve"=w177, "Nstep"=w89, "Max Gain"=w152, "Amp of Q curve"=w178, "Step Width (MHz)"=w134, "Center Freq (MHz)"=w135) -> ("Start"=w201:i32, "Array"=w202:dbl[])
        n98 = global read "Global 2.vi" "Real/Quad Q curve"() -> (w176:bool)
        n99 = To Double Precision Float(number=w159) -> (double precision float=w132:dbl)
        n100 = Array Subset "Array Subset"(array=w202, index=w201, length=w89) -> (w187:dbl[])
        n101 = property on="Property Node" class="VI"(reference=w108, error in=w107) -> ("Exec.State"=w110:T2)  [unwired: 2 out]
        n102 = global read "Global 2.vi" "AutoTune"() -> (w174:bool)
        n103 = Select(t=w187, s=w176, f=w185) -> (s? t:f=w102:dbl[])
        n104 = Not(x=w174) -> (.not. x?=w188:bool)
        n105 = Equal?(x=2, y=w110) -> (x = y?=→"He readback":bool)
        n106 = Not(x="Stop Run") -> (.not. x?=w77:bool)
        n107 = Greater?(x=w150, y=7.5) -> (0:w191:bool)
        n108 = Not(x=w191) -> (.not. x?=w170:bool)
        "RF level OK" <- w170
        n109 = global write "Global 2.vi" "RF OK"(w170) -> ()
        n110 = case shown="True" w77 {
          frame False {
          }
          frame True {
            n111 = stacked-sequence {
              frame #0 {
                n112 = Wait (ms)(milliseconds to wait=100) -> ()  [unwired: 1 out]
              }
              frame #1 {
                n113 = Stop() -> ()  [unwired: 1 in]
              }
            }
          }
        }
        n114 = global read "Global 2.vi" "Amp of Q curve"() -> (w123:dbl)
        n115 = To Double Precision Float(number=w159) -> (double precision float=w154:dbl)
        n116 = global read "Global 2.vi" "RemovePed"() -> (w175:bool)
        n117 = Equal To 0?(x=w88) -> (x = 0?=w158:bool)
        n118 = call "RemoveQandP.vi"("Subtract Ped?"=w175, "Qcurve"=w102, "Raw data"=w119) -> ("Ped L-R"=w195:dbl, "Corrected data"=w143:dbl[], "Ped Offfset"=w165:dbl)
        "Pedestal (V)" <- w165
        n119 = global write "Global 2.vi" "Pedestal Offset"(w165) -> ()
        n120 = global read "Global 2.vi" "Gauss Fit"() -> (w173:bool)
        n121 = global write "Global 2.vi" "Sample RMS (V)"(w136) -> ()
        n122 = Get Date/Time In Seconds() -> (seconds since 1Jan1904=w86:timestamp)
        n123 = global write "Global 2.vi" "Temperature (C)"(w131) -> ()
        n124 = Array Max & Min "Array Max"(array=w143) -> (max value=w127:dbl)  [unwired: 3 out]
        n125 = call-poly <vilib>:"Power Spectrum.vi"("X"=w119) -> ("Power Spectrum"=w148:dbl[])  [unwired: 1 out]
        n126 = global read "Global 2.vi" "Calib Constant"() -> (w122:dbl)
        n127 = Absolute Value ("Abs Value")(x=w195) -> (abs(x)=w196:dbl)
        n128 = Negate(x=w195) -> (-x=w166:dbl)
        "Pedestal Diff (V)" <- w166
        n129 = call "FitData.vi"("Fit?"=w173, "Fmax"=w190, "Fmin"=w138, "Yarray"=w143) -> ("Peak Area (mV-MHz)"=w125:dbl, "Center Freq (MHz)"=w169:dbl, "NMR Graph + Fit"=w167:cluster{cluster{dbl, "Numeric":dbl}[]}[])  [unwired: 2 out]
        "Peak area (V-MHz)" <- w125
        "Peak center (MHz)" <- w169
        n130 = Build Array (concatenate) "Header + Data"(w135, w134, w133, w132, w131, w130, w129, w128, w118, w125, w123, w122, w120, w115, w114, w119) -> (w82:dbl[])
        n131 = global write "Global 2.vi" "Peak area (mV-MHz)"(w125) -> ()
        n132 = Square Root(x=w148) -> (sqrt(x)=w144:dbl[])
        "FFT Vrms" <- w144
        n133 = global write "Global 2.vi" "NMR Graph + Fit"(w167) -> ()
        n134 = call "SaveData.vi"("Array"=w82, "Save Data to File"=TRUE, "Ext time (sec)"=w81) -> ()  [unwired: 1 out]
        n135 = call "SaveTune.vi"("Array"=w82, "Save Data to File"="Save Tune", "Ext time (sec)"=w81) -> ()  [unwired: 1 out]
        n136 = global write "Global 2.vi" "Pedestal Difference"(w166) -> ()
        n137 = global write "Global 2.vi" "Pedestal Diff (V)"(w166) -> ()
        n138 = Select(t=w119, s=w140, f=w144) -> (s? t:f=w100:dbl[])
        n139 = Format Date/Time String(time format string (%c)="%c", seconds (now)=w86) -> (date/time string=→"Date / Time":string)  [unwired: 1 in]
        n140 = feedback #2 "Feedback Node"() -> (w157:dbl[])  [unwired: 1 in]
        n141 = case shown="False" w158 {
          tunnel: w100 -> [w229 w231]
          tunnel: [w228 w231] -> w155
          tunnel: w157 -> [w230 _]
          frame False {
            # "Sum sweeps"
            n142 = Add(x=w230, y=w229) -> (x+y=w228:dbl[])
          }
          frame True {
            # "Initialize"
          }
        }
        n143 = feedback-in #2(w155) -> ()
        n144 = Divide(x=w155, y=w154) -> (x/y=w101:dbl[])
        n145 = Multiply(x=w122, y=w127) -> (x*y=w126:dbl)
        n146 = Select(t=0.1, s=w152, f=0.01) -> (s? t:f=w160:dbl)
        n147 = Multiply(x=w125, y=w122) -> (x*y=w124:dbl)
        n148 = Greater?(x=w196, y=w160) -> (0:w162:bool)
        n149 = call "ADCok.vi"("PedOK"=w162, "Array"=w119, "Vmax-1/2"=w156) -> ("Vmin"=w182:dbl, "ADC voltages OK"=w172:bool, "Allok"=w189:bool)
        "ADC volts OK" <- w172
        n150 = Multiply(x=w182, y=10.0) -> (x*y=w180:dbl)
        n151 = call "Autozero.vi"("Vmin (V)"=w180, "IFoffset (V)"=w150, "Enable"=w188, "Max Gain"=w152) -> ()
        n152 = global read "Global - Pressure & Flow.vi" "Task3 Temperature"() -> (→"He temp (K)":dbl)
        n153 = global read "Global - Pressure & Flow.vi" "Task3 Pressure"() -> (→"He press (torr)":dbl)
        n154 = And(x=w189, y=w161) -> (x .and. y?=w197:bool)
        n155 = case shown="False" w189 {
          frame False {
            # "All OK"
            n156 = property on="Raw NMR Graph / Ave" class="WFGraph (strict)"("Active Plot"=0, "Plot.Plot Color"=u32 13145856) -> ()  [unwired: 2 in, 2 out]
          }
          frame True {
            # "Bad data"
            n157 = property on="Raw NMR Graph / Ave" class="WFGraph (strict)"("Active Plot"=0, "Plot.Plot Color"=u32 16711680) -> ()  [unwired: 2 in, 2 out]
          }
        }
        n158 = Not(x=w162) -> (.not. x?=w171:bool)
        "Pedestal volts OK" <- w171
        n159 = global write "Global 2.vi" "Peak center (MHz)"(w169) -> ()
        n160 = Select(t=w124, s=w173, f=w126) -> (s? t:f=w168:dbl)
        "Peak amp (V)" <- w168
        n161 = global read "Global 2.vi" "Subtract Q curve"() -> (w103:bool)
        n162 = case shown="False" w103 {
          tunnel: w100 -> [w223 w227]
          tunnel: [w222 w226] -> w104
          tunnel: w102 -> [_ w225]
          tunnel: w87 -> [w221 w224]
          frame False {
            n163 = Build Array(w223, w221) -> (w222:dbl[][])
          }
          frame True {
            n164 = Build Array(w227, w224, w225) -> (w226:dbl[][])
          }
        }
        n165 = Select(t=w138, s=w140, f=0.0) -> (s? t:f=w137:dbl)
        n166 = Select(t=w134, s=w140, f=1.0) -> (s? t:f=w141:dbl)
        n167 = global write "Global 2.vi" "Pedestal OK"(w171) -> ()
        n168 = global write "Global 2.vi" "ADC volts OK"(w172) -> ()
        n169 = case shown="True" w197 {
          tunnel: [w236 -99.0] -> w198
          tunnel: w168 -> [w236 _]
          frame False {
            # "Data OK"
          }
          frame True {
            # "flag it bad"
          }
        }
        n170 = global write "Global 2.vi" "Peak Height"(w168) -> ()
        n171 = global write "Global 2.vi" "Peak amp (V)"(w168) -> ()
        n172 = Bundle(w137, "Step Width (MHz)"=w141, w104) -> (→"Raw NMR Graph / Ave":cluster{dbl, "Step Width (MHz)":dbl, dbl[][]})  [unwired: 1 in]
        n173 = Build Array (concatenate) "Build Array"(w137, w141, w101) -> (w151:dbl[])
      }
      n174 = call "DataQA.vi"("Quality cuts"=w65, "Data In"=w73) -> ("Data Out"=w72:dbl[])
      n175 = global read "Global 2.vi" "Save Data to File"() -> (w58:bool)
      n176 = call <vilib>:"Std Deviation and Variance.vi"("X"=w72) -> ("mean"=w63:dbl, "standard deviation"=w53:dbl)  [unwired: 1 in, 1 out]
      "Peak mean (V)" <- w63
      n177 = Multiply(x=w53, y=1000.0) -> (x*y=→"Peak RMS (mV)":dbl)
      n178 = call "PeakHisto.vi"("Data Out"=w72) -> ("XY Graph"=w61:cluster{"Y":dbl[], "Y":dbl[]}[])
      "Peak Height Distribution" <- w61
      n179 = global write "Global 2.vi" "Peak Height Distribution"(w61) -> ()
      n180 = global write "Global 2.vi" "Peak mean (V)"(w63) -> ()
      n181 = call "SaveDataAve.vi"("Array"=w59, "Save Data to File"=w58) -> ()  [unwired: 1 in, 1 out]
      n182 = Array Size(array=w72) -> (size(s)=w62:i32)
      "# Good Spectra" <- w62
      n183 = global write "Global 2.vi" "# Good Spectra"(w62) -> ()
      n184 = Divide(x=w63, y=w53) -> (x/y=w64:dbl)
      "S/N" <- w64
      n185 = global write "Global 2.vi" "S/N"(w64) -> ()
    }
    frame #2 {
      n186 = property on="Property Node" class="VI"(reference=w282, error in=w281) -> (reference out=w284:refnum<vi>, error out=w283:errorcluster, "Exec.State"=w286:T2)
      n187 = Equal?(x=2, y=w286) -> (x = y?=w285:bool)
      n188 = case shown="True" w285 {
        tunnel: w284 -> [_ w293]
        tunnel: w283 -> [_ w292]
        frame False {
        }
        frame True {
          # "Stop MKS routine and close panel if running"
          # "Add simple error handling\nfor VI operations"
          n189 = invoke on="Invoke Node" class="VI" method="Abort VI"(reference=w293, error in=w292) -> (reference out=w290:refnum<vi>, error out=w289:errorcluster)  [unwired: 1 in, 1 out]
          n190 = property on="Property Node" class="VI"(reference=w290, error in=w289, "Front Panel Window:Open"=FALSE) -> (error out=w288:errorcluster)  [unwired: 1 out]
          n191 = call <vilib>:"Simple Error Handler.vi"("type of dialog (OK msg:1)"=1, "error in (no error)"=w288) -> ()  [unwired: 3 in, 5 out]
        }
      }
    }
  }
